vi "Delete Subscription.vi"(8 "error in (no error)":errorcluster, 11 "Subscription":refnum<class "Subscription.lvclass">) -> (0 "error out":errorcluster)   [LabVIEW 2015, in "NI_AWS_SNS.lvlib" / "Subscription.lvclass"]
uses:
  Subscription.lvclass
  Core/ARN/ARN.lvclass
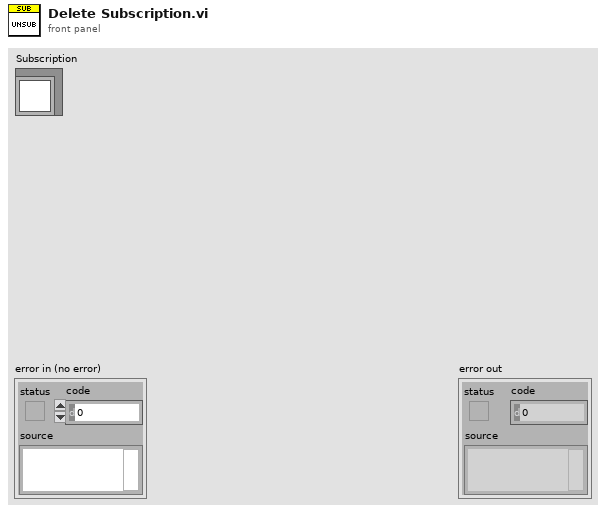
[diagram p1: front panel]
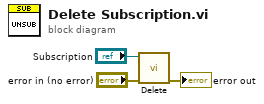
[diagram p0: block diagram]
diagram:
  n1 = call "Delete.vi"("error in (no error)"="error in (no error)", "ARN in"="Subscription") -> ("error out"=→"error out":errorcluster)  [unwired: 9 in]
